vi "rename to VIPT.vi"() -> (0 "error out":errorcluster)   [LabVIEW 2013]
panel:
  in  "error in (no error)":errorcluster
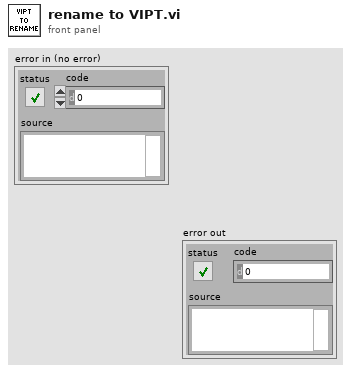
[diagram p1: front panel]
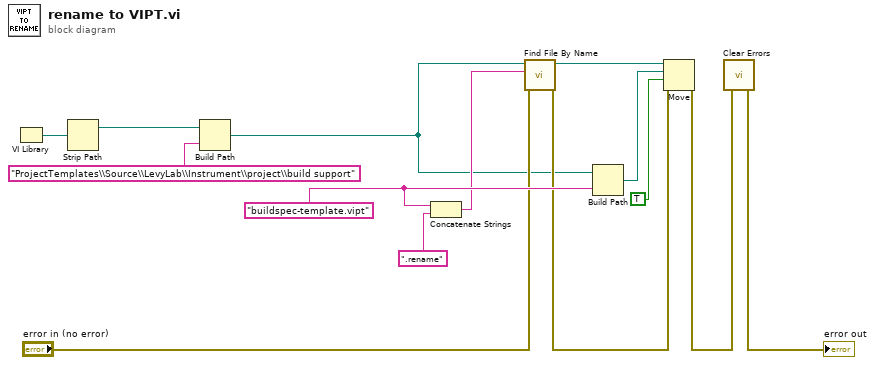
[diagram p0: block diagram]
diagram:
  w10 = "buildspec-template.vipt" ("name or relative path")
  n1 = VI Library() -> (path=w9:path)
  n2 = Strip Path(path=w9) -> (stripped path=w8:path)  [unwired: 1 out]
  n3 = Build Path(base path=w8, name or relative path="ProjectTemplates\\Source\\LevyLab\\Instrument\\project\\build support") -> (appended path=w1:path)
  n4 = Concatenate Strings(w10, ".rename" ("name or relative path")) -> (w2:string)
  n5 = call "Find File By Name.vi"("error in (no error)"="error in (no error)", "File Name"=w2, "Folder Path"=w1) -> ("error out"=w5:errorcluster, "File Path"=w7:path)  [unwired: 7 in]
  n6 = Build Path(base path=w1, name or relative path=w10) -> (appended path=w13:path)
  n7 = Move(source path=w7, error in=w5, 9:TRUE ("overwrite (F)"), 10:w13) -> (error out=w12:errorcluster)  [unwired: 1 in, 2 out]
  n8 = call <vilib>:"Clear Errors.vi"("error in (no error)"=w12) -> ("error out"=→"error out":errorcluster)  [unwired: 5 in, 1 out]
